vi "Button Detect.vi"(7 "State":enum16{"Initialize", "Compare"}(ring), 8 "error in (no error)":errorcluster, 9 "CAN Frame [Write]":cluster{"Identifier":u32, "Data Bytes":u8[]} {"Data Bytes" format="%x"; "Identifier" format="%x"}, 10 "output cluster":T1) -> (0 "error out":errorcluster, 2 "Freq":dbl, 4 "State Out":T2, 5 "CAN Frame [Write] Out":T3 {"payload" format="%x"; "timestamp" format="%<%I:%M:%S%8u %p\n%x>T"; "identifier" format="%x"})   [LabVIEW 2015]
uses:
  <vilib>/Stratom, Inc/X-CAN for myRIO (API)/X-CAN Class/Type Definitions/CANFrame.ctl
  Control/State.ctl
  <vilib>/Stratom, Inc/X-CAN for myRIO (API)/X-CAN Class/X-CAN.lvclass
panel:
  # "Since myRIO is a real-time device, and the event structure doesn't work on real-time device.\nThus this vi detect which button is pressed by comparing the current button state with the last state."
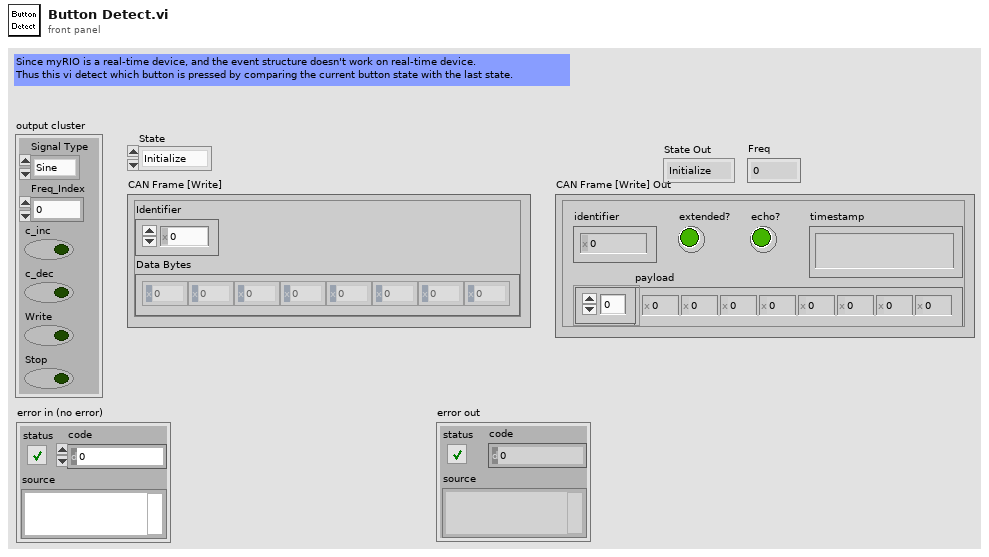
[diagram p1: front panel]
types:
  T1 = cluster{"Signal Type":enum16{"Sine", "Square", "Triangle"}, "Freq_Index":u8, "c_inc":bool, "c_dec":bool, "Write":bool, "Stop":bool}
  T2 = typedef "State.ctl" = enum16{"Initialize", "Idle", "Write", "Stop"}
  T3 = typedef "X-CAN.lvclass/CANFrame.ctl" = cluster{"identifier":u32, "extended?":bool, "echo?":bool, "payload":u8[], "timestamp":timestamp}
  T4 = cluster{"Signal Type":bool, "Freq_Index":bool, "c_inc":bool, "c_dec":bool, "Write":bool, "Stop":bool}
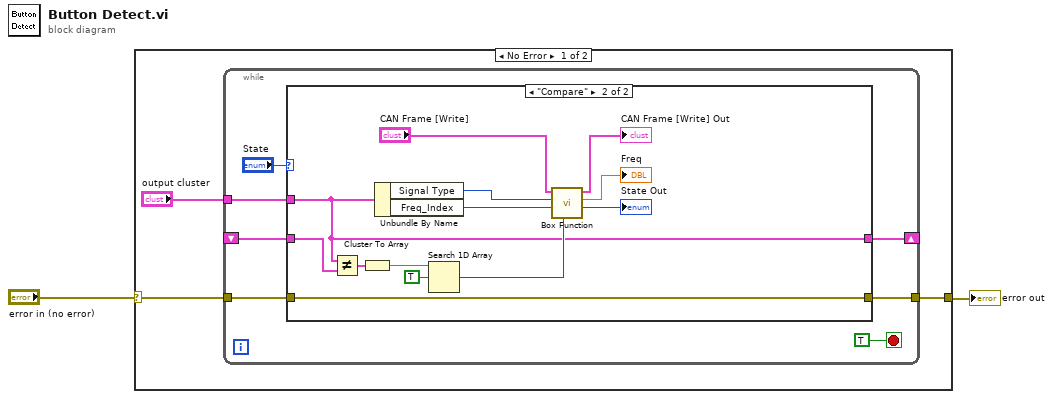
[diagram p0: block diagram]
diagram:
  n1 = case shown="No Error" "error in (no error)" {
    selector: "error in (no error)" -> [w5 w28]
    tunnel: [w4 w28] -> w1
    frame No Error {
      n2 = while {
        shift-right: [w8] -> _
        shift-left: _ -> [w10]
        tunnel: "output cluster" -> [w9]
        tunnel: w5 -> [w7]
        tunnel: [w6] -> w4
        stop <- TRUE stop-if-true
        n3 = case shown="\"Compare\"" "State" {
          tunnel: w10 -> [_ w25]
          tunnel: [w14 w24] -> w8
          tunnel: w9 -> [w14 w24]
          tunnel: w7 -> [w13 w15]
          tunnel: [w13 w15] -> w6
          frame "Initialize", Default {
          }
          frame "Compare" {
            n4 = Not Equal?(x=w24, y=w25) -> (x != y?=w20:T4)
            n5 = Cluster To Array(cluster=w20) -> (array=w27:bool[])
            n6 = Unbundle By Name(w24) -> ("Signal Type"=w17:enum16{"Sine", "Square", "Triangle"}, "Freq_Index"=w18:u8)
            n7 = Search 1D Array(1D array=w27, element=TRUE) -> (index of element=w26:i32)  [unwired: 1 in]
            n8 = call "Box Function.vi"("Index"=w26, "Freq Index"=w18, "Signal Type"=w17, "CAN Frame [Write] In"="CAN Frame [Write]") -> ("State"=→"State Out":T2, "Freq"=→"Freq":dbl, "CAN Frame [Write]"=→"CAN Frame [Write] Out":T3)  [unwired: 5 in]
          }
        }
      }
    }
    frame Error {
    }
  }
  "error out" <- w1
